vi "Tosca-Purge Pupillometry Data.vi"(0 "Path":path, 11 "error in (no error)":errorcluster) -> (15 "error out":errorcluster)   [LabVIEW 2020]
uses:
  epl-vi-lib/TCP VIs/TCP Params.ctl
  Tosca-Globals.vi
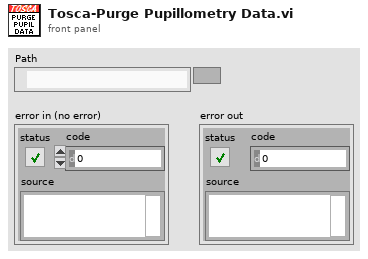
[diagram p1: front panel]
types:
  T1 = enum16{"big-endian, network order", "native, host order", "little-endian"}
  T2 = typedef "TCP Params.ctl" = cluster{"IP Address":string, "Port":i32}
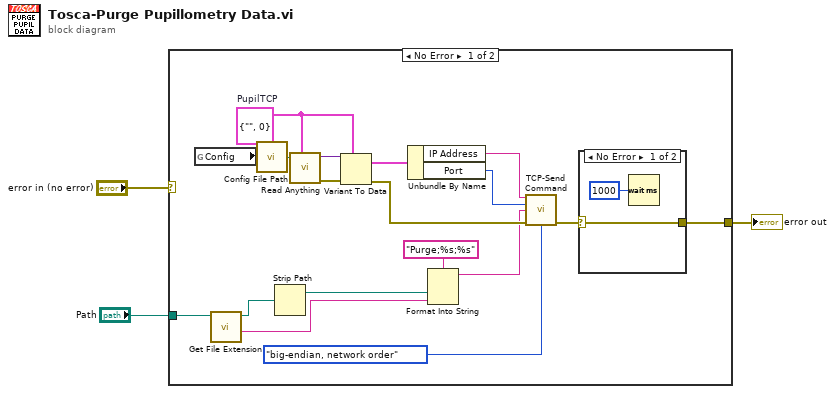
[diagram p0: block diagram]
diagram:
  n1 = case shown="No Error" "error in (no error)" {
    selector: "error in (no error)" -> [_ w25]
    tunnel: [w7 w25] -> w2
    tunnel: "Path" -> [w15 _]
    frame No Error {
      w20 = T2 {"IP Address"="", "Port"=0}  # PupilTCP
      n2 = global read "Tosca-Globals.vi" "Config"() -> (w5:string)
      n3 = call <vilib>:"Get File Extension.vi"("file"=w15) -> ("filename without extension"=w11:string, "dup file"=w13:path)  [unwired: 6 in, 3 out]
      n4 = call "Config File Path.vi"("AppName"=w5) -> ("Default config file name"=w21:path)
      n5 = Strip Path(path=w13) -> (stripped path=w12:path)  [unwired: 1 out]
      n6 = call "Read Anything.vi"("Type of Anything"=w20, "Path (dialog)"=w21) -> ("Error Out"=w18:errorcluster, "Anything"=w19:variant)  [unwired: 7 in, 1 out]
      n7 = Variant To Data(error in=w18, type=w20, Variant=w19) -> (data=w17:T2, error out=w16:errorcluster)
      n8 = Unbundle By Name(w17) -> ("IP Address"=w10:string, "Port"=w9:i32)
      n9 = Format Into String(format string="Purge;%s;%s", w12, w11) -> (resulting string=w6:string)  [unwired: 2 in, 1 out]
      n10 = call "TCP-Send Command.vi"("PXI Address"=w10, "Port"=w9, "Command"=w6, "error in (no error)"=w16, "byte order"=T1."big-endian, network order") -> ("error out"=w8:errorcluster)  [unwired: 10 in]
      n11 = case shown="No Error" w8 {
        selector: w8 -> [w22 w24]
        tunnel: [w22 w24] -> w7
        frame No Error {
          n12 = Wait (ms)(milliseconds to wait=u32 1000) -> ()  [unwired: 1 out]
        }
        frame Error {
        }
      }
    }
    frame Error {
    }
  }
  "error out" <- w2
